vi "Read Connections.vi"(9 "Wire in":refnum<class "Wire.lvclass">) -> (3 "Wire out":refnum<class "Wire.lvclass">, 4 "Connections":T1[](array[typedef]))   [LabVIEW 2014, in "Wire.lvclass"]
uses:
  Wire.lvclass
  ConnectionsTD.ctl
  Terminal/Terminal.lvclass
  Wire.lvclass/Wire.ctl
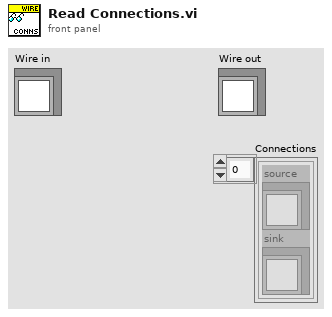
[diagram p1: front panel]
types:
  T1 = typedef "ConnectionsTD.ctl" = cluster{"source":refnum<class "Terminal.lvclass">, "sink":refnum<class "Terminal.lvclass">}
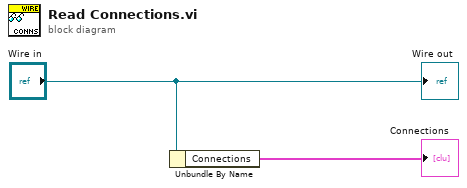
[diagram p0: block diagram]
diagram:
  n1 = Unbundle By Name("Wire in") -> ("Connections"=→"Connections":T1[])
  "Wire out" <- "Wire in"
